vi "New Multi-pattern Matcher.vi"(8 "error in (no error)":errorcluster, 11 "Library Directory":path) -> (0 "error out":errorcluster, 3 "New MultiPattern Matcher":refnum<class "MultiPattern Matcher.lvclass">)   [LabVIEW 2013, in "MultiPattern Matcher.lvclass"]
uses:
  MultiPattern Matcher.lvclass
  MultiPattern Matcher.lvclass/MultiPattern Matcher.ctl
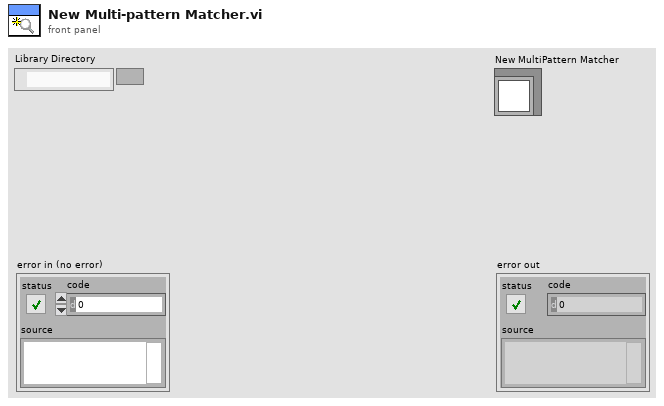
[diagram p1: front panel]
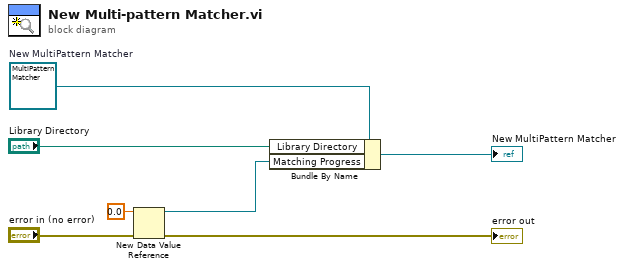
[diagram p0: block diagram]
diagram:
  w4 = refnum<class "MultiPattern Matcher.lvclass"> refnum  # New MultiPattern Matcher
  n1 = New Data Value Reference(data value=0.0, error in="error in (no error)") -> (data value reference=w3:refnum<data-value>, error out=→"error out":errorcluster)
  n2 = Bundle By Name(cluster=w4, "Library Directory"="Library Directory", "Matching Progress"=w3) -> (→"New MultiPattern Matcher":refnum<class "MultiPattern Matcher.lvclass">)
